vi "user initialization.vi"(8 "error in":errorcluster, 10 "configuration in":refnum<class "control module configuration.lvclass">, 11 "fixed channel runtime in":refnum<class "RTResourceUtilitzation runtime.lvclass">) -> (0 "error out":errorcluster, 3 "fixed channel runtime out":refnum<class "RTResourceUtilitzation runtime.lvclass">)   [LabVIEW 2014, in "RTResourceUtilitzation runtime.lvclass"]
uses:
  RTResourceUtilitzation runtime.lvclass
  <vilib>/NI/DCAF/Tag Editor Core/control module/configuration/control module configuration.lvclass
  RTResourceUtilitzation runtime.lvclass/RTResourceUtilitzation runtime.ctl
  <vilib>/NI/DCAF/Tag Editor Core/control module/runtime/control module runtime.lvclass
  <vilib>/nisyscfg/nisyscfg.lvlib
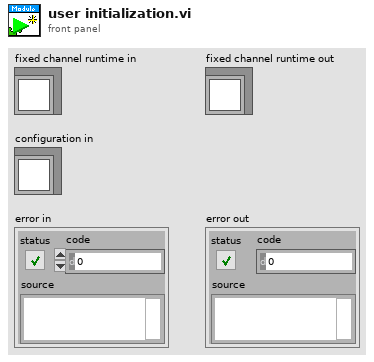
[diagram p1: front panel]
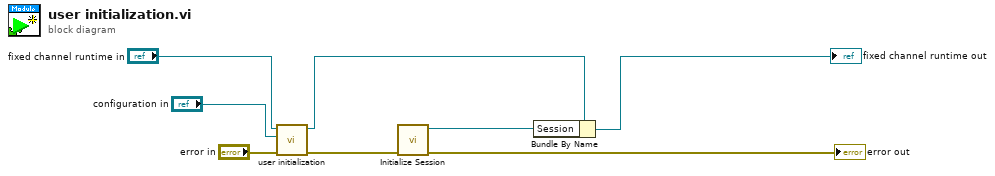
[diagram p0: block diagram]
diagram:
  n1 = call-parent "user initialization.vi"("error in"="error in", "configuration in"="configuration in", "fixed channel runtime in"="fixed channel runtime in") -> ("error out"=w5:errorcluster, "fixed channel runtime out"=w2:refnum<class "RTResourceUtilitzation runtime.lvclass">)  [unwired: 7 in]
  n2 = call <vilib>:"Initialize Session.vi"("error in (no error)"=w5) -> ("error out"=→"error out":errorcluster, "Session out"=w3:refnum<k21>)  [unwired: 9 in]
  n3 = Bundle By Name(cluster=w2, "Session"=w3) -> (→"fixed channel runtime out":refnum<class "RTResourceUtilitzation runtime.lvclass">)
